vi "Insight Example VI.vi"   [LabVIEW 2012]
uses:
  <vilib>/Rock Robotics/SystemInterfaces/Typedef/FPGA_TypedefDigitalModule.ctl
  Loop Count Global.vi
types:
  T1 = enum16{"FOUR_ZONES", "ONE_ZONE_TWO_LINES", "TWO_ZONES_ONE_LINE"}
  T2 = typedef "FPGA_TypedefDigitalModule.ctl" = enum16{"Digital Module 1", "Digital Module 2"}
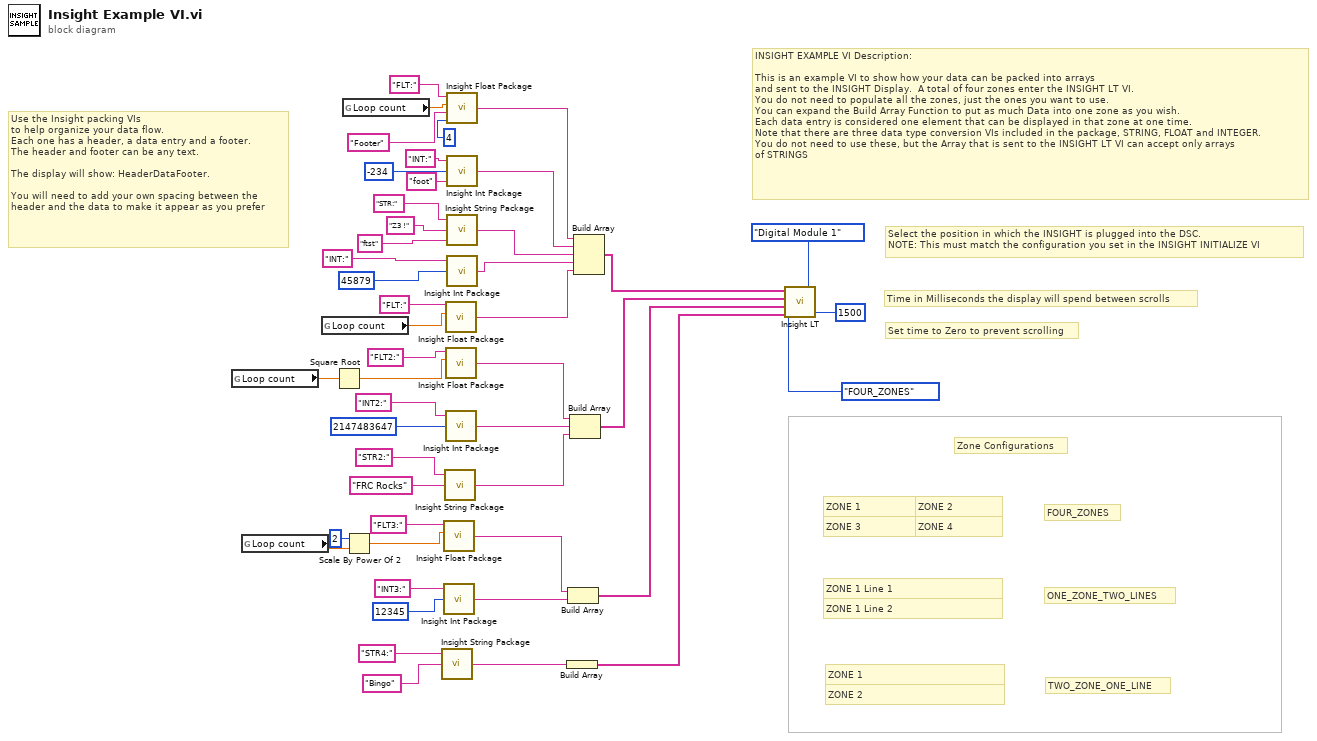
[diagram p0: block diagram]
diagram:
  # "Set time to Zero to prevent scrolling"
  # "Use the Insight packing VIs\nto help organize your data flow.\nEach one has a header, a data entry and a footer.\nThe header and footer can be any text.\n\nThe display will show: HeaderDataFooter.\n\nYou will need to add your own spacing between the \nheader and the data to make it appear as you prefer"
  # "TWO_ZONE_ONE_LINE"
  # "ONE_ZONE_TWO_LINES"
  # "FOUR_ZONES"
  # "Zone Configurations"
  # "ZONE 4"
  # "ZONE 2"
  # "ZONE 3"
  # "ZONE 1"
  # "ZONE 1 Line 2"
  # "ZONE 1 Line 1"
  # "ZONE 2"
  # "ZONE 1"
  # "Time in Milliseconds the display will spend between scrolls"
  # "Select the position in which the INSIGHT is plugged into the DSC.\nNOTE: This must match the configuration you set in the INSIGHT INITIALIZE VI"
  # "INSIGHT EXAMPLE VI Description:\n\nThis is an example VI to show how your data can be packed into arrays\nand sent to the INSIGHT Display.  A total of four zones enter the INSIGHT LT VI. \nYou do not need to populate all the zones, just the ones you want to use.\nYou can expand the Build Array Function to put as much Data into one zone as you wish.\nEach data entry is considered one element that can be displayed in that zone at one time.\nNote that there are three data type conversion VIs included in the package, STRING, FLOAT and INTEGER.\nYou do not need to use these, but the Array that is sent to the INSIGHT LT VI can accept only arrays\nof STRINGS"
  n1 = global read "Loop Count Global.vi" "Loop count"() -> (w26:dbl)
  n2 = global read "Loop Count Global.vi" "Loop count"() -> (w22:dbl)
  n3 = global read "Loop Count Global.vi" "Loop count"() -> (w7:dbl)
  n4 = Square Root(x=w26) -> (sqrt(x)=w25:dbl)
  n5 = global read "Loop Count Global.vi" "Loop count"() -> (w47:dbl)
  n6 = Scale By Power Of 2(n=i16 2, x=w22) -> (x*2^n=w23:dbl)
  n7 = call "Insight String Package.vi"("String"="Bingo", "Header"="STR4:") -> ("resulting string"=w12:string)  [unwired: 1 in]
  n8 = call "Insight Float Package.vi"("Float"=w23, "Header"="FLT3:") -> ("resulting string"=w18:string)  [unwired: 2 in]
  n9 = call "Insight Int Package.vi"("Int32"=12345, "Header"="INT3:") -> ("resulting string"=w17:string)  [unwired: 1 in]
  n10 = call "Insight String Package.vi"("String"="FRC Rocks", "Header"="STR2:") -> ("resulting string"=w34:string)  [unwired: 1 in]
  n11 = call "Insight Float Package.vi"("Float"=w7, "Header"="FLT:") -> ("resulting string"=w5:string)  [unwired: 2 in]
  n12 = call "Insight Float Package.vi"("Float"=w25, "Header"="FLT2:") -> ("resulting string"=w32:string)  [unwired: 2 in]
  n13 = call "Insight Int Package.vi"("Int32"=2147483647, "Header"="INT2:") -> ("resulting string"=w33:string)  [unwired: 1 in]
  n14 = call "Insight Float Package.vi"("Decimal Places"=4, "Footer"="Footer", "Float"=w47, "Header"="FLT:") -> ("resulting string"=w39:string)
  n15 = call "Insight Int Package.vi"("Footer"="foot", "Int32"=-234, "Header"="INT:") -> ("resulting string"=w38:string)
  n16 = call "Insight String Package.vi"("Footer"="ftst", "String"="Z3 !", "Header"="STR:") -> ("resulting string"=w37:string)
  n17 = call "Insight Int Package.vi"("Int32"=45879, "Header"="INT:") -> ("resulting string"=w6:string)  [unwired: 1 in]
  n18 = Build Array(w12) -> (w13:string[])
  n19 = Build Array(w18, w17) -> (w14:string[])
  n20 = Build Array(w32, w33, w34) -> (w24:string[])
  n21 = Build Array(w39, w38, w37, w6, w5) -> (w36:string[])
  n22 = call "Insight LT.vi"("Scroll Timing"=1500, "ZONE \nCONFIGURATION"=T1."FOUR_ZONES" ("ZONE \nCONFIGURATION"), "Digital Module"=FPGA_TypedefDigitalModule."Digital Module 1", "Zone 4 Data"=w13, "Zone 3 Data"=w14, "Zone 2 Data"=w24, "Zone 1 Data"=w36) -> ()
